vi "半周期测量_单点.vi"() -> ()   [LabVIEW 2013]
uses:
  <userlib>/ArtDAQ/_SubVI/ArtDAQ_CreateCISemiPeriodChan.vi
  <userlib>/ArtDAQ/_SubVI/ArtDAQ_Read Counter DBL 1Samp.vi
panel:
  out "数据s":dbl
  in  "计数器":string="Dev1/ctr0"
  in  "最小测量值":dbl=1e-06 format="%0.6f"
  in  "最大测量值":dbl=10.0 format="%0.6f"
  out "错误输出":errorcluster
  # "通道属性"
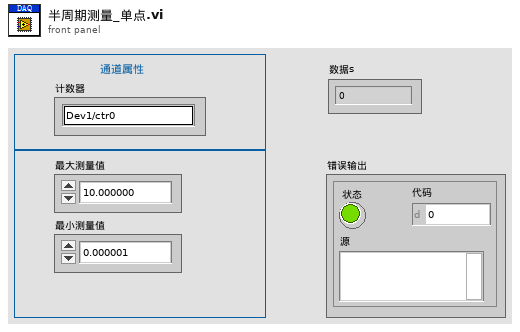
[diagram p1: front panel]
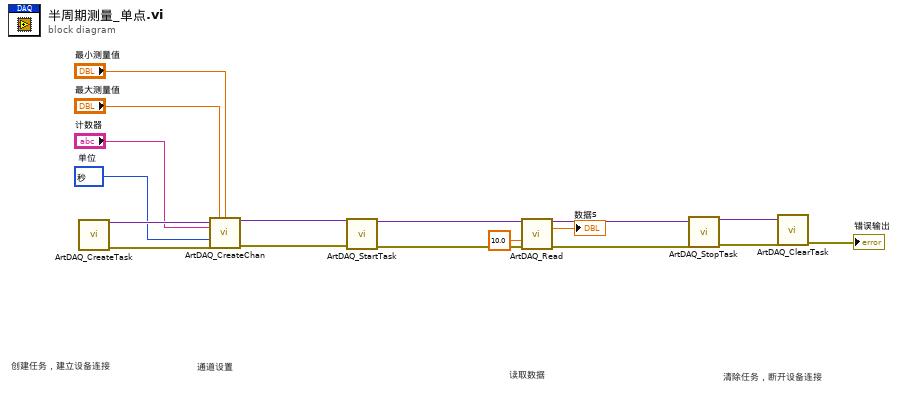
[diagram p0: block diagram]
diagram:
  w1 = 10364 items=["秒"=10364, "时钟滴答"=10304, "来自自定义换算"=10065]  # 单位
  # "清除任务，断开设备连接"
  # "读取数据"
  # "通道设置"
  # "创建任务，建立设备连接"
  n1 = call <userlib>:"ArtDAQ_CreateTask.vi"() -> ("任务句柄"=w17:variant, "错误输出"=w16:errorcluster)  [unwired: 14 in]
  n2 = call-poly <userlib>:"ArtDAQ_CreateChan.vi"("任务句柄"=w17, "最大值"="最大测量值", "最小值"="最小测量值", "计数器"="计数器", "单位"=w1, "错误输入"=w16) -> ("任务句柄"=w5:variant, "错误输出"=w4:errorcluster)  [unwired: 8 in]
  n3 = call <userlib>:"ArtDAQ_StartTask.vi"("任务句柄"=w5, "错误输入"=w4) -> ("任务句柄"=w9:variant, "错误输出"=w8:errorcluster)  [unwired: 12 in]
  n4 = call-poly <userlib>:"ArtDAQ_Read.vi"("任务句柄"=w9, "超时s"=10.0 ("Timeout"), "错误输入"=w8) -> ("任务句柄"=w14:variant, "数据"=→"数据s":dbl, "错误输出"=w12:errorcluster)  [unwired: 10 in]
  n5 = call <userlib>:"ArtDAQ_StopTask.vi"("任务句柄"=w14, "错误输入"=w12) -> ("任务句柄"=w13:variant, "错误输出"=w11:errorcluster)  [unwired: 12 in]
  n6 = call <userlib>:"ArtDAQ_ClearTask.vi"("任务句柄"=w13, "错误输入"=w11) -> ("错误输出"=→"错误输出":errorcluster)  [unwired: 13 in]
